vi "MT Rician Selective Fading profile (Gans).vi"(0 "profile length (samples)":i32=1000, 1 "rician parameter K (dB)":dbl format="%.2f", 2 "number of paths":i32=1, 5 "sampling frequency (Hz)":dbl=1.0 format="%.2f", 7 "doppler spread (Hz)":dbl=0.01 format="%.2p", 9 "seed in (0xFFFFFFFF)":i32=-1 format="%.0x", 11 "error in (no error)":errorcluster, 12 "fading variance":dbl=1.0 format="%.2f", 13 "reset? (T)":bool=TRUE) -> (4 "fading profile":cdb[][](array[numeric]), 10 "seed out":i32 format="%.0x", 15 "error out":errorcluster)   [LabVIEW 2020, in "niDMT.lvlib"]
doc: "This polymorphic instance generates a Rician selective-fading profile for the multipath channel. The envelope for the first path statistically obeys the Rician distribution, while the envelope for the remaining paths obey the Raleigh distribution implemented using the Gans model."
uses:
  <vilib>/addons/Modulation/niDMT.lvlib
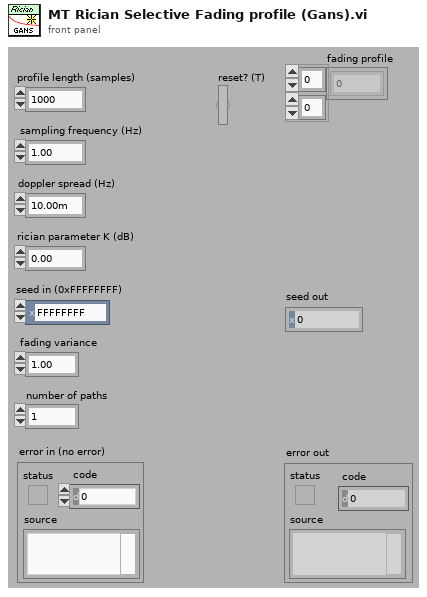
[diagram p1: front panel]
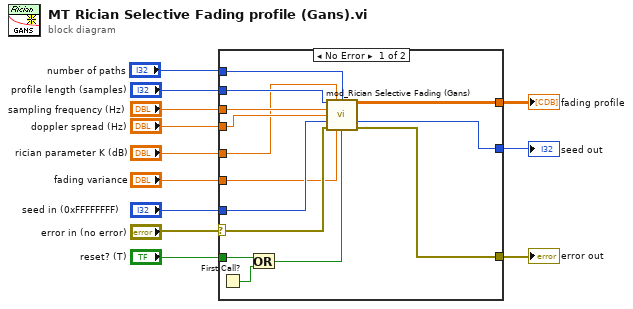
[diagram p0: block diagram]
diagram:
  n1 = case shown="No Error" "error in (no error)" {
    selector: "error in (no error)" -> [w21 w27]
    tunnel: "profile length (samples)" -> [w24 _]
    tunnel: [w26 _] -> w2
    tunnel: [w25 w27] -> w11
    tunnel: "sampling frequency (Hz)" -> [w23 _]
    tunnel: "doppler spread (Hz)" -> [w22 _]
    tunnel: "reset? (T)" -> [w20 _]
    tunnel: "seed in (0xFFFFFFFF)" -> [w17 _]
    tunnel: "rician parameter K (dB)" -> [w16 _]
    tunnel: "fading variance" -> [w15 _]
    tunnel: [w14 _] -> w3
    tunnel: "number of paths" -> [w13 _]
    frame No Error {
      n2 = First Call?() -> (First Call?: T/F=w19:bool)
      n3 = Or(x=w20, y=w19) -> (x .or. y?=w18:bool)
      n4 = call <vilib>:"mod_Rician Selective Fading (Gans).vi"("profile length (samples)"=w24, "rician parameter K (dB)"=w16, "number of paths"=w13, "sampling frequency (Hz)"=w23, "doppler spread (Hz)"=w22, "seed in (0xFFFFFFFF)"=w17, "error in (no error)"=w21, "fading variance"=w15, "reset? (T)"=w18) -> ("Rician Fading profile"=w26:cdb[][], "next seed"=w14:i32, "error out"=w25:errorcluster)  [unwired: 4 out]
    }
    frame Error {
    }
  }
  "error out" <- w11
  "seed out" <- w3
  "fading profile" <- w2
